vi "Overlay.vi"(8 "error in (no error)":errorcluster, 11 "Vision in":refnum<class "Vision.lvclass">) -> (0 "error out":errorcluster, 3 "Vision out":refnum<class "Vision.lvclass">)   [LabVIEW 2019, in "Vision.lvlib" / "Vision.lvclass"]
uses:
  Vision.lvclass
  Vision.lvclass/Vision.ctl
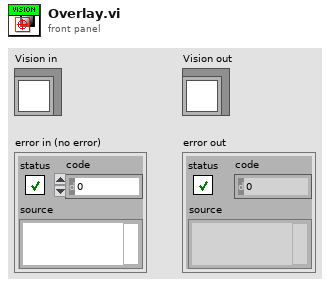
[diagram p1: front panel]
types:
  T1 = cluster{"Left":i32, "Top":i32, "Right":i32, "Bottom":i32}
  T2 = cluster{"Contour Type":u32, "ROI Type":u32, "Points":i32[]}[]
  T3 = typedef "IMAQ Image.ctl" = refnum<image>
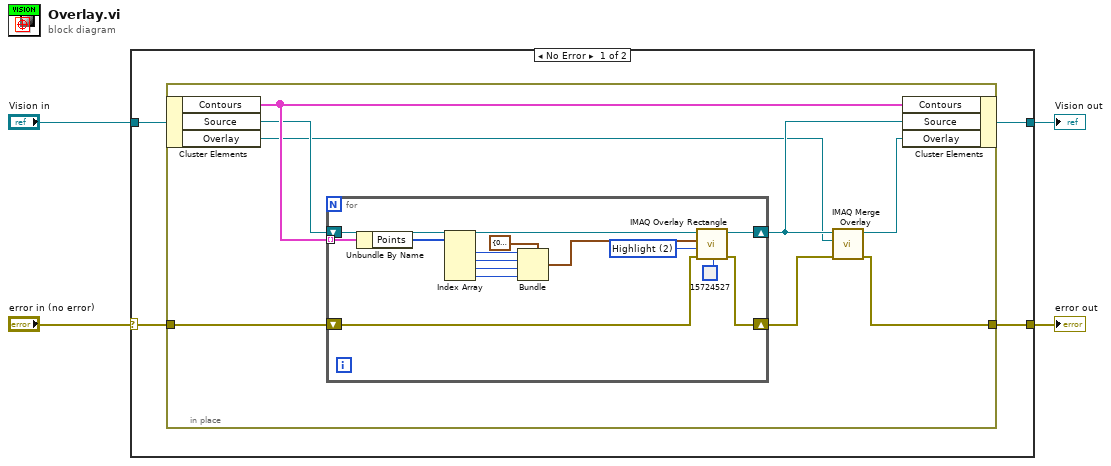
[diagram p0: block diagram]
diagram:
  n1 = case shown="No Error" "error in (no error)" {
    selector: "error in (no error)" -> [w7 w32]
    tunnel: [w6 w32] -> w3
    tunnel: [w5 w31] -> w1
    tunnel: "Vision in" -> [w8 w31]
    frame No Error {
      n2 = in-place {
        in-place-border: w7 -> [w15]
        in-place-border: [w9] -> w6
        n3 = in-place-cluster #1(w8) -> ("Contours"=w16:T2, "Source"=w14:T3, "Overlay"=w11:T3)
        n4 = for {
          shift-right: [w29] -> w12
          shift-left: w14 -> [w30]
          tunnel: w16 -> [w28] mode=indexing
          shift-right: [w17] -> w13
          shift-left: w15 -> [w18]
          w27 = u32 2 items=["Frame", "Fill", "Highlight"] ("Drawing Mode (Frame)")
          n5 = Unbundle By Name(w28) -> ("Points"=w25:i32[])
          n6 = Index Array(array=w25) -> (element #1=w24:i32, element #2=w23:i32, element #3=w22:i32, element #4=w21:i32)  [unwired: 4 in]
          n7 = Bundle(cluster=T1 {"Left"=0, "Top"=0, "Right"=0, "Bottom"=0} ("Rectangle"), "Left"=w24, "Top"=w23, "Right"=w22, "Bottom"=w21) -> (w20:T1)
          n8 = call "IMAQ Overlay Rectangle"("Color"=u32 15724527, "error in (no error)"=w18, "Drawing Mode (Frame)"=w27, "Rectangle"=w20, "Image"=w30) -> ("error out"=w17:errorcluster, "Image Out"=w29:T3)  [unwired: 5 in]
        }
        n9 = call "IMAQ Merge Overlay"("error in (no error)"=w13, "Image Dst"=w11, "Image Src"=w12) -> ("error out"=w9:errorcluster, "Image Dst Out"=w10:T3)  [unwired: 7 in]
        n10 = in-place-cluster #1("Contours"=w16, "Source"=w12, "Overlay"=w10) -> (w5:refnum<class "Vision.lvclass">)
      }
    }
    frame Error {
    }
  }
  "error out" <- w3
  "Vision out" <- w1
